vi "Get motor position.vi"(9 "Data from port":string, 10 "Motor2 in":i32, 11 "Motor1 in":i32) -> (2 "Motor2 out":i32, 3 "Motor1 out":i32)   [LabVIEW 2020]
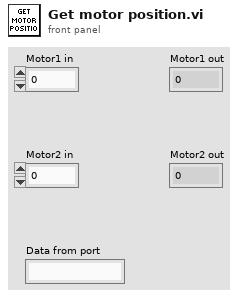
[diagram p1: front panel]
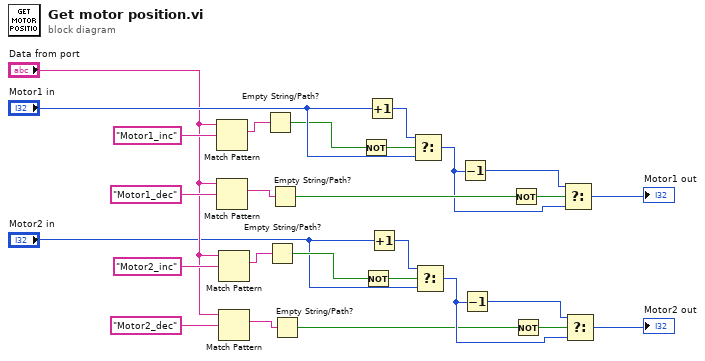
[diagram p0: block diagram]
diagram:
  n1 = Match Pattern(string="Data from port", regular expression="Motor1_inc") -> (match substring=w26:string)  [unwired: 1 in, 3 out]
  n2 = Match Pattern(string="Data from port", regular expression="Motor1_dec") -> (match substring=w19:string)  [unwired: 1 in, 3 out]
  n3 = Match Pattern(string="Data from port", regular expression="Motor2_inc") -> (match substring=w5:string)  [unwired: 1 in, 3 out]
  n4 = Match Pattern(string="Data from port", regular expression="Motor2_dec") -> (match substring=w11:string)  [unwired: 1 in, 3 out]
  n5 = Empty String/Path?(string/path=w26) -> (empty?=w22:bool)
  n6 = Empty String/Path?(string/path=w5) -> (empty?=w8:bool)
  n7 = Empty String/Path?(string/path=w19) -> (empty?=w18:bool)
  n8 = Empty String/Path?(string/path=w11) -> (empty?=w12:bool)
  n9 = Not(x=w22) -> (.not. x?=w27:bool)
  n10 = Not(x=w8) -> (.not. x?=w4:bool)
  n11 = Increment(x="Motor1 in") -> (x+1=w23:i32)
  n12 = Increment(x="Motor2 in") -> (x+1=w7:i32)
  n13 = Select(t=w23, s=w27, f="Motor1 in") -> (s? t:f=w16:i32)
  n14 = Select(t=w7, s=w4, f="Motor2 in") -> (s? t:f=w14:i32)
  n15 = Decrement(x=w16) -> (x-1=w17:i32)
  n16 = Decrement(x=w14) -> (x-1=w13:i32)
  n17 = Not(x=w18) -> (.not. x?=w20:bool)
  n18 = Not(x=w12) -> (.not. x?=w10:bool)
  n19 = Select(t=w17, s=w20, f=w16) -> (s? t:f=→"Motor1 out":i32)
  n20 = Select(t=w13, s=w10, f=w14) -> (s? t:f=→"Motor2 out":i32)
